vi "Begin.vi"(7 "Simulated?":bool, 8 "error in (no error)":errorcluster, 9 "Solenoids":T1, 10 "Pneumatics Control Module (9)":u8=9, 11 "Pneumatics in":refnum<class "Pneumatics.lvclass">) -> (0 "error out":errorcluster, 3 "Pneumatics out":refnum<class "Pneumatics.lvclass">)   [LabVIEW 2018, in "Pneumatics control.lvlib" / "Pneumatics.lvclass"]
uses:
  Pneumatics.lvclass
  TypeDefs/Solenoids.ctl
  Solenoids/Solenoids.lvclass
  Pneumatics.lvclass/Pneumatics.ctl
  <vilib>/Rock Robotics/WPI/Utilities/WPI_GetSetVariantRefNum.vi
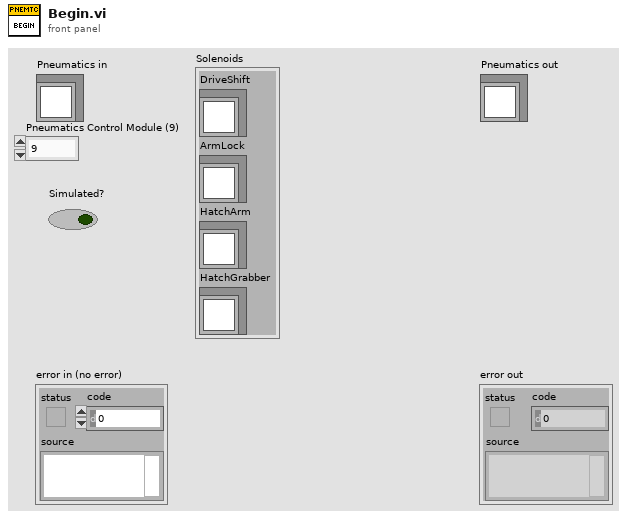
[diagram p1: front panel]
types:
  T1 = typedef "Pneumatics control.lvlib/Pneumatics.lvclass/Solenoids.ctl" = cluster{"DriveShift":refnum<class "Solenoids.lvclass">, "ArmLock":refnum<class "Solenoids.lvclass">, "HatchArm":refnum<class "Solenoids.lvclass">, "HatchGrabber":refnum<class "Solenoids.lvclass">}
  T2 = typedef "WPI_CompressorDevRef.ctl" = cluster{"DevStatus":errorcluster, "Pneumatics Control Module":u8}
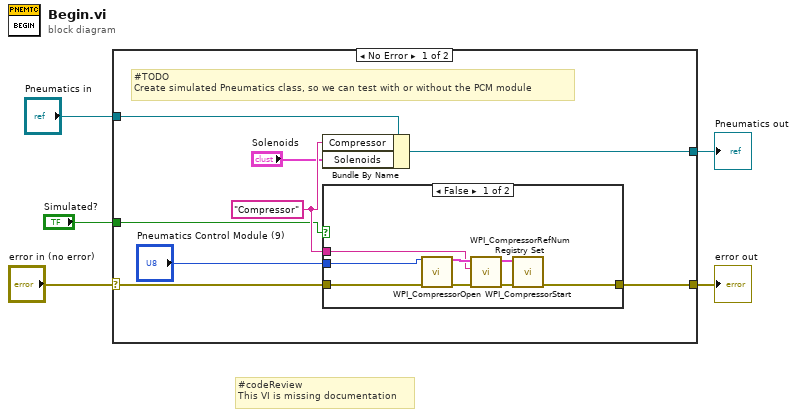
[diagram p0: block diagram]
diagram:
  # "#codeReview\nThis VI is missing documentation"
  n1 = case shown="No Error" "error in (no error)" {
    selector: "error in (no error)" -> [w8 w24]
    tunnel: [w10 w24] -> w4
    tunnel: [w12 w23] -> w2
    tunnel: "Pneumatics in" -> [w13 w23]
    tunnel: "Simulated?" -> [w6 _]
    frame No Error {
      w11 = "Compressor" ("refnum name")
      # "#TODO\nCreate simulated Pneumatics class, so we can test with or without the PCM module"
      n2 = Bundle By Name(cluster=w13, "Compressor"=w11, "Solenoids"="Solenoids") -> (w12:refnum<class "Pneumatics.lvclass">)
      n3 = case shown="False" w6 {
        tunnel: w11 -> [w17 _]
        tunnel: [w16 w22] -> w10
        tunnel: w8 -> [w15 w22]
        tunnel: "Pneumatics Control Module (9)" -> [w14 _]
        frame False {
          n4 = call <vilib>:"WPI_CompressorOpen.vi"("Pneumatics Control Module (0)"=w14, "error in (no error)"=w15) -> ("CompressorDevRef"=w21:T2, "error out"=w19:errorcluster)  [unwired: 12 in]
          n5 = call <vilib>:"WPI_CompressorRefNum Registry Set.vi"("error in (no error)"=w19, "refnum name"=w17, "CompressorDevRef"=w21) -> ("error out"=w18:errorcluster, "CompressorDevRef"=w20:T2)  [unwired: 7 in]
          n6 = call <vilib>:"WPI_CompressorStart.vi"("error in (no error)"=w18, "CompressorDevRef"=w20) -> ("error out"=w16:errorcluster)  [unwired: 8 in, 1 out]
        }
        frame True {
          # "If simulated, then do not open the compressor"
        }
      }
    }
    frame Error {
    }
  }
  "error out" <- w4
  "Pneumatics out" <- w2
